vi "ShooterWhileLoop.vi"() -> (7 "Disc Fired":bool)   [LabVIEW 2012]
uses:
  Robot Global Data.vi
panel:
  in  "Boolean":bool
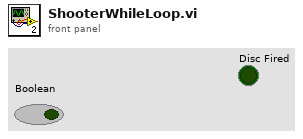
[diagram p1: front panel]
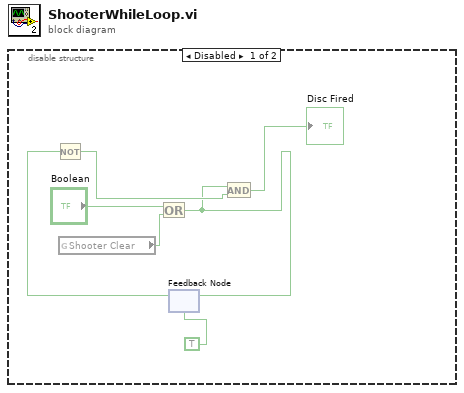
[diagram p0: block diagram]
diagram:
  n1 = disable-structure shown="Disabled" {
    frame Disabled {
      n2 = global read "Robot Global Data.vi" "Shooter Clear"() -> (w7:bool)
      n3 = Or(x="Boolean", y=w7) -> (x .or. y?=w4:bool)
      n4 = feedback #1(TRUE) -> (w3:bool)
      n5 = Not(x=w3) -> (.not. x?=w5:bool)
      n6 = feedback-in #1(w4) -> ()
      n7 = And(x=w4, y=w5) -> (x .and. y?=→"Disc Fired":bool)
    }
    frame Enabled {
    }
  }
